vi "Create All Message Queues.vi"(8 "error in (no error)":errorcluster) -> (0 "error out":errorcluster, 3 "Message Queues":T1)   [LabVIEW 2015, in "a Message Queue.lvlib"]
doc: "This VI creates and initializes all the message queues for your application. If your application requires more than one message queue, right-click the \"Message Queues\" constant above and select Open Type Def. Add the new Message Queue(s) to the type definition, then initialize them in this VI."
uses:
  a Message Queue.lvlib
  Exercise 3-2/Course Project/support/Message Queue/All Message Queues.ctl
  Exercise 3-2/Course Project/support/Message Queue/Message Cluster.ctl
  Enqueue Message (Single).vi
  Exercise 3-2/Course Project/support/Message Queue/Message Queue.lvlib
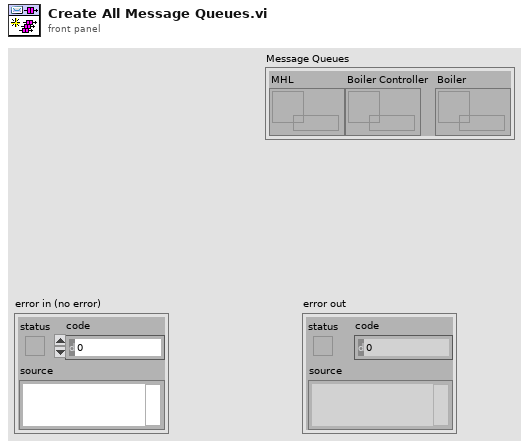
[diagram p1: front panel]
types:
  T1 = typedef "Message Queue.lvlib/All Message Queues.ctl" = cluster{"MHL":refnum<queue>, "Boiler Controller":refnum<queue>, "Boiler ":refnum<queue>}
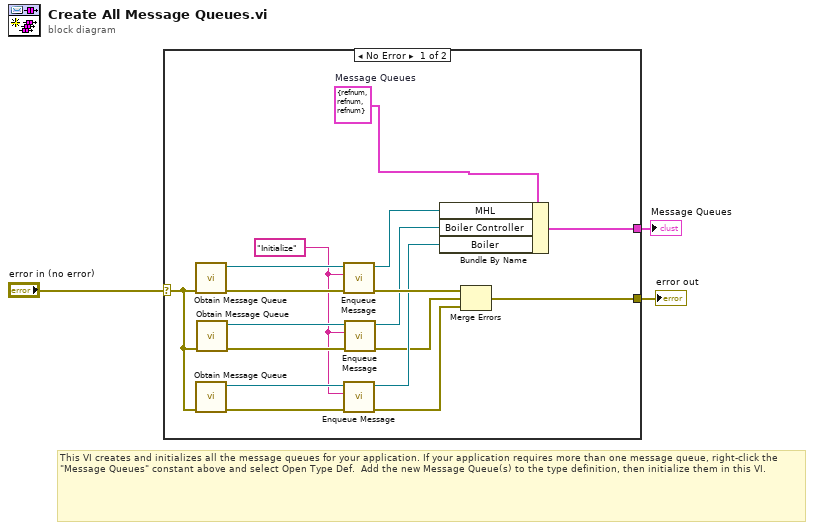
[diagram p0: block diagram]
diagram:
  # "This VI creates and initializes all the message queues for your application. If your application requires more than one message queue, right-click the \"Message Queues\" constant above and select Open Type Def.  Add the new Message Queue(s) to the type definition, then initialize them in this VI."
  n1 = case shown="No Error" "error in (no error)" {
    selector: "error in (no error)" -> [w12 w21]
    tunnel: [w7 w21] -> w3
    tunnel: [w19 _] -> w1
    frame No Error {
      w4 = T1 {"MHL"=refnum, "Boiler Controller"=refnum, "Boiler "=refnum}  # Message Queues
      w11 = "Initialize" ("Message")
      n2 = call "Obtain Message Queue.vi"("error in (no error)"=w12) -> ("error out"=w18:errorcluster, "Message Queue"=w17:refnum<queue>)  [unwired: 9 in]
      n3 = call "Obtain Message Queue.vi"("error in (no error)"=w12) -> ("error out"=w14:errorcluster, "Message Queue"=w13:refnum<queue>)  [unwired: 9 in]
      n4 = call "Obtain Message Queue.vi"("error in (no error)"=w12) -> ("error out"=w15:errorcluster, "Message Queue"=w16:refnum<queue>)  [unwired: 9 in]
      n5 = call-poly "Enqueue Message.vi"("error in (no error)"=w18, "Message"=w11, "Message Queue"=w17) -> ("error out"=w20:errorcluster, "dup Message Queue"=w10:refnum<queue>)  [unwired: 7 in]
      n6 = call-poly "Enqueue Message.vi"("error in (no error)"=w14, "Message"=w11, "Message Queue"=w13) -> ("error out"=w5:errorcluster, "dup Message Queue"=w8:refnum<queue>)  [unwired: 7 in]
      n7 = call-poly "Enqueue Message.vi"("error in (no error)"=w15, "Message"=w11, "Message Queue"=w16) -> ("error out"=w6:errorcluster, "dup Message Queue"=w9:refnum<queue>)  [unwired: 7 in]
      n8 = Bundle By Name(cluster=w4, "MHL"=w10, "Boiler Controller"=w9, "Boiler"=w8) -> (w19:T1)
      n9 = Merge Errors(w20, w6, w5) -> (w7:errorcluster)
    }
    frame Error {
    }
  }
  "error out" <- w3
  "Message Queues" <- w1
